vi "DN4_1Darray2DDT.vi"(1 "Array":dbl[](array[numeric])) -> (0 "Dynamic Data Type":dynamicdata(graph))   [LabVIEW 2009]
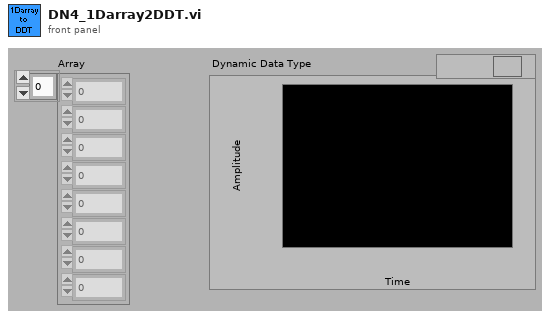
[diagram p1: front panel]
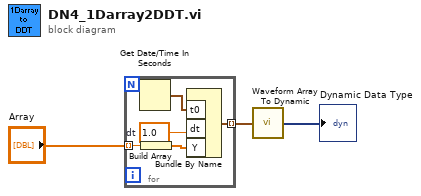
[diagram p0: block diagram]
diagram:
  n1 = for {
    tunnel: "Array" -> [w8] mode=indexing
    tunnel: [w6] -> w3 mode=indexing
    w5 = 1.0  # dt
    n2 = Get Date/Time In Seconds() -> (seconds since 1Jan1904=w4:timestamp)
    n3 = Build Array(w8) -> (w7:dbl[])
    n4 = Bundle By Name("t0"=w4, "dt"=w5, "Y"=w7) -> (w6:waveform(dbl))  [unwired: 1 out]
  }
  n5 = call <vilib>:"Waveform Array To Dynamic.vi"("Input"=w3) -> ("Output"=→"Dynamic Data Type":dynamicdata)  [unwired: 4 out]
